vi "SP Update Marker Plot Labels.vi"(5 "CH Control":T1={"Trace Orientation"=enum."Overlay", "Frequency"={"Change Frequency"=FALSE, "Start"=500.0, "Stop"=1500.0, "Units"=enum."MHz"}, "Markers"=[], "Traces"=[]} {"Traces"."Reference" format="%#.2g"; "Traces"."Display Data" items=["Data", "Memory", "Data/Memory"]; "Traces"."Format" items=["Log Mag", "Phase", "Expanded Phase", "Delay", "Smith", "Polar", "Lin Mag", "SWR", "Loss", "Real", "Imaginary"]; "Traces"."Scale" min=0.001 step=1.0 format="%#.2g"; "Traces"."Position" min=0.0 max=10.0; "Frequency"."Stop" format="%.3g"; "Frequency"."Start" format="%.3g"}, 7 "Plot References":refnum<vi>[](array[refnum]), 8 "error in (no error)":errorcluster, 11 "Plot Ref":refnum<vi>) -> (0 "error out":errorcluster)   [LabVIEW 2011]
uses:
  TypeDefs/SP Display Plot Controls Cluster.ctl
  TypeDefs/SP Frequency Units.ctl
  TypeDefs/SP Marker Cluster.ctl
  TypeDefs/SP Marker Type.ctl
  TypeDefs/SP Display Trace Controls.ctl
  TypeDefs/SP Display Format.ctl
  TypeDefs/SP Display Data.ctl
  TypeDefs/SP Plot Cluster Object.ctl
panel:
  # "Div"
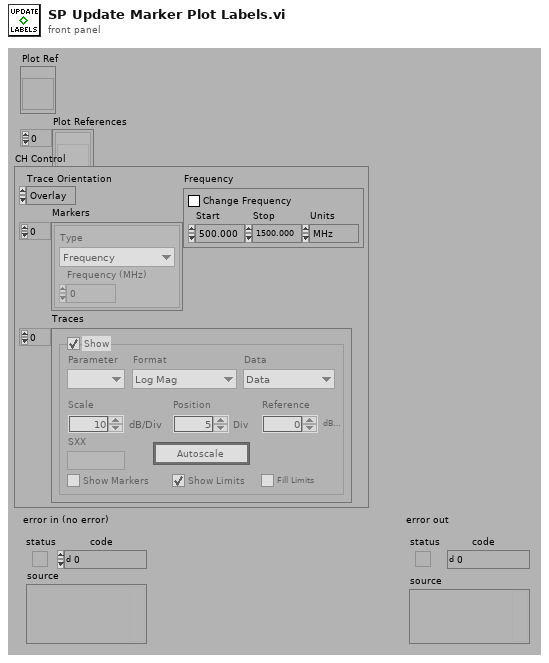
[diagram p1: front panel]
types:
  T1 = typedef "SP Display Plot Controls Cluster.ctl" = cluster{"Trace Orientation":enum32{"Overlay", "Split"}, "Frequency":cluster{"Change Frequency":bool, "Start":dbl, "Stop":dbl, "Units":T2}, "Markers":T3[], "Traces":T5[]}
  T2 = typedef "SP Frequency Units.ctl" = enum16{"Hz", "kHz", "MHz", "GHz", "Points"}
  T3 = typedef "SP Marker Cluster.ctl" = cluster{"Type":T4, "Frequency (MHz)":dbl}
  T4 = typedef "SP Marker Type.ctl" = enum16{"Frequency", "Trace Maximum", "Trace Minimum", "Limit Maximum", "Limit Minimum"}
  T5 = typedef "SP Display Trace Controls.ctl" = cluster{"Trace On":bool, "Measure":i32, "Format":T6, "Autoscale":bool, "Reference":dbl, "\nRefUnit":string, "Position":dbl, "Scale":dbl, "ScaleUnit":string, "LimitOn":bool, "LimitFill":bool, "Display Data":T7, "Show Markers":bool, "SXX":string}
  T6 = typedef "SP Display Format.ctl" = i32
  T7 = typedef "SP Display Data.ctl" = u16
  T8 = typedef "SP Plot Cluster Object.ctl" = enum16{"Plot", "CH Reference", "CH Label", "Start Label", "Stop Label", "Units Label", "Selected?", "CH Markers"}
  T9 = typedef "SP Channel Data.ctl" = cluster{"Graph Ref":refnum<vi>, "Data":cluster{"Data":cluster{"X":dbl[], "Y":dbl[]}, "Index":i32}, "ULimits":cluster{"Data":cluster{"X":dbl[], "Y":dbl[]}, "Index":i32}[], "LLimits":cluster{"Data":cluster{"X":dbl[], "Y":dbl[]}, "Index":i32}[]}
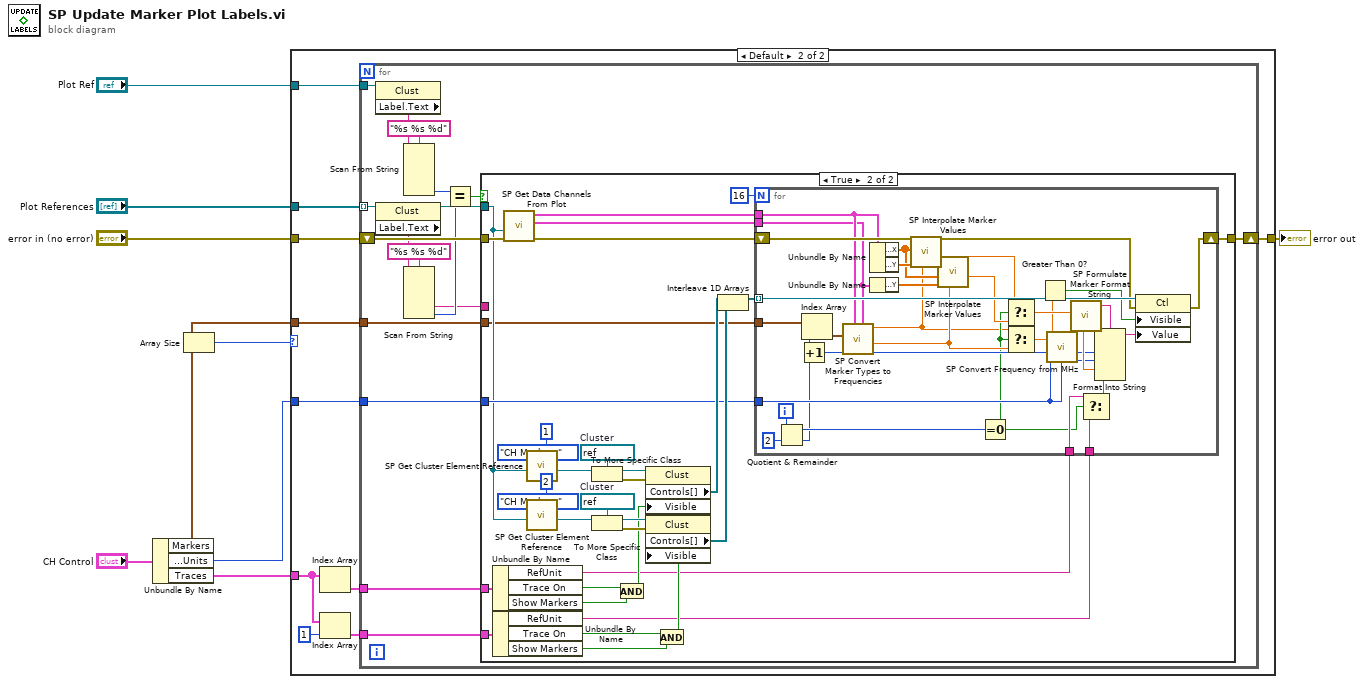
[diagram p0: block diagram]
diagram:
  n1 = Unbundle By Name("CH Control") -> ("Markers"=w4:T3[], "Frequency.Units"=w5:T2, "Traces"=w1:T5[])
  n2 = Array Size(array=w4) -> (size(s)=w3:i32)
  n3 = case shown="Default" w3 {
    tunnel: "Plot References" -> [_ w18]
    tunnel: "error in (no error)" -> [w10 w20]
    tunnel: [w10 w19] -> w9
    tunnel: "Plot Ref" -> [_ w17]
    tunnel: w5 -> [_ w16]
    tunnel: w4 -> [_ w15]
    tunnel: w1 -> [_ w11]
    frame 9.. {
      # "If there are already 4 markers, don't add anymore."
    }
    frame Default {
      n4 = Index Array(array=w11) -> (element=w12:T5)  [unwired: 1 in]
      n5 = Index Array(array=w11, index=1) -> (element=w13:T5)
      n6 = for {
        tunnel: w18 -> [w35] mode=indexing
        tunnel: w17 -> [w31]
        shift-right: [w36] -> w19
        shift-left: w20 -> [w37]
        tunnel: w12 -> [w24]
        tunnel: w13 -> [w23]
        tunnel: w16 -> [w22]
        tunnel: w15 -> [w21]
        n7 = property class="Clust"(reference=w31) -> ("Label.Text"=w29:string)  [unwired: 1 in, 2 out]
        n8 = property class="Clust"(reference=w35) -> (reference out=w34:refnum<vi>, "Label.Text"=w32:string)  [unwired: 1 in, 1 out]
        n9 = Scan From String(format string="%s %s %d", input string=w29) -> (output 3=w28:i32)  [unwired: 2 in, 8 out]
        n10 = Scan From String(format string="%s %s %d", input string=w32) -> (output 2=w25:string, output 3=w27:i32)  [unwired: 2 in, 7 out]
        n11 = Equal?(x=w28, y=w27) -> (x = y?=w26:bool)
        n12 = case shown="True" w26 {
          tunnel: w37 -> [w38 w44]
          tunnel: [w38 w72] -> w36
          tunnel: w34 -> [_ w42]
          tunnel: w25 -> [_ _]
          tunnel: w24 -> [_ w49]
          tunnel: w23 -> [_ w48]
          tunnel: w22 -> [_ w47]
          tunnel: w21 -> [_ w41]
          frame False {
          }
          frame True {
            w63 = refnum<vi> refnum  # Cluster
            w60 = refnum<vi> refnum  # Cluster
            n13 = Unbundle By Name(w49) -> ("RefUnit"=w45:string, "Trace On"=w53:bool, "Show Markers"=w52:bool)
            n14 = Unbundle By Name(w48) -> ("RefUnit"=w46:string, "Trace On"=w51:bool, "Show Markers"=w50:bool)
            n15 = call "SP Get Data Channels From Plot.vi"("error in (no error)"=w44, "Plot Ref"=w42) -> ("error out"=w43:errorcluster, "CH 2"=w40:T9, "CH 1"=w39:T9)  [unwired: 7 out]
            n16 = call "SP Get Cluster Element Reference.vi"("Channel"=i8 1, "Element"=SP_Plot_Cluster_Object."CH Markers", "Plot Reference"=w42) -> ("Element Reference"=w71:refnum<vi>)  [unwired: 6 out]
            n17 = call "SP Get Cluster Element Reference.vi"("Channel"=i8 2, "Element"=SP_Plot_Cluster_Object."CH Markers", "Plot Reference"=w42) -> ("Element Reference"=w64:refnum<vi>)  [unwired: 6 out]
            n18 = To More Specific Class(target class=w60, reference=w71) -> (specific class reference=w69:refnum<vi>, error out=w68:errorcluster)  [unwired: 1 in]
            n19 = To More Specific Class(target class=w63, reference=w64) -> (specific class reference=w66:refnum<vi>, error out=w67:errorcluster)  [unwired: 1 in]
            n20 = And(x=w53, y=w52) -> (x .and. y?=w56:bool)
            n21 = property class="Clust"(reference=w69, error in=w68, "Visible"=w56) -> ("Controls[]"=w59:refnum<vi>[])  [unwired: 2 out]
            n22 = And(x=w51, y=w50) -> (x .and. y?=w57:bool)
            n23 = property class="Clust"(reference=w66, error in=w67, "Visible"=w57) -> ("Controls[]"=w58:refnum<vi>[])  [unwired: 2 out]
            n24 = Interleave 1D Arrays(w59, w58) -> (w54:refnum<vi>[])
            n25 = for {
              N: 16 -> [_]
              shift-right: [w100] -> w72
              shift-left: w43 -> [w93]
              tunnel: w54 -> [w101] mode=indexing
              tunnel: w47 -> [w86]
              tunnel: w46 -> [w92]
              tunnel: w45 -> [w91]
              tunnel: w41 -> [w89]
              tunnel: w40 -> [w77]
              tunnel: w39 -> [w78]
              i -> [w96]
              n26 = Quotient & Remainder(x=w96, y=2) -> (x-y*floor(x/y)=w97:i32, floor(x/y)=w80:i32)
              n27 = Increment(x=w80) -> (x+1=w88:i32)
              n28 = Index Array(array=w89, index=w80) -> (element=w79:T3)
              n29 = call "SP Convert Marker Types to Frequencies.vi"("CH 2"=w77, "CH 1"=w78, "Marker"=w79) -> ("CH2 Frequency"=w76:dbl, "CH1 Frequency"=w73:dbl)  [unwired: 5 out]
              n30 = Unbundle By Name(w78) -> ("Data.Data.X"=w81:dbl[], "Data.Data.Y"=w84:dbl[])
              n31 = Unbundle By Name(w77) -> ("Data.Data.Y"=w85:dbl[])
              n32 = call "SP Interpolate Marker Values.vi"("Marker Value"=w73, "Y Values"=w84, "X Values"=w81) -> ("Interpolated Y Value"=w82:dbl)  [unwired: 8 out]
              n33 = call "SP Interpolate Marker Values.vi"("Marker Value"=w76, "Y Values"=w85, "X Values"=w81) -> ("Interpolated Y Value"=w83:dbl)  [unwired: 8 out]
              n34 = Equal To 0?(x=w97) -> (x = 0?=w75:bool)
              n35 = Select(t=w82, s=w75, f=w83) -> (s? t:f=w90:dbl)
              n36 = Select(t=w73, s=w75, f=w76) -> (s? t:f=w74:dbl)
              n37 = Greater Than 0?(x=w74) -> (x > 0?=w94:bool)
              n38 = call "SP Convert Frequency from MHz.vi"("Units"=w86, "Frequency (MHz)"=w74) -> ("Converted Frequency"=w87:dbl)  [unwired: 1 in, 8 out]
              n39 = call "SP Formulate Marker Format String.vi"("X Value"=w87, "Y Value"=w90) -> ("Format String"=w95:string)  [unwired: 7 out]
              n40 = Select(t=w91, s=w75, f=w92) -> (s? t:f=w98:string)
              n41 = Format Into String(format string=w95, w88, w86, w90, w98) -> (resulting string=w102:string)  [unwired: 2 in, 1 out]
              n42 = property class="Ctl"(reference=w101, error in=w93, "Visible"=w94, "Value"=w102) -> (error out=w100:errorcluster)  [unwired: 1 out]
            }
          }
        }
      }
    }
  }
  "error out" <- w9
